vi "update hydrolysis feeding.vi"(7 "number_timestamps":i32, 8 "error in (no error)":errorcluster, 9 "amount":string, 10 "time":string, 11 "hydrolysis_specfile":string) -> (0 "error out":errorcluster)   [LabVIEW 2019, in "libFileFunctions.lvlib"]
doc: "void update_hydrolysis_feeding(const char* hydrolysis_specfile, double time[], double amount[], int number_timestamps);"
uses:
  libFileFunctions.lvlib
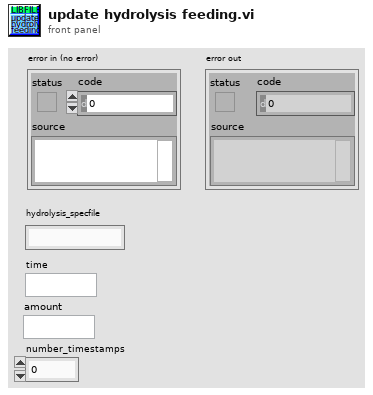
[diagram p1: front panel]
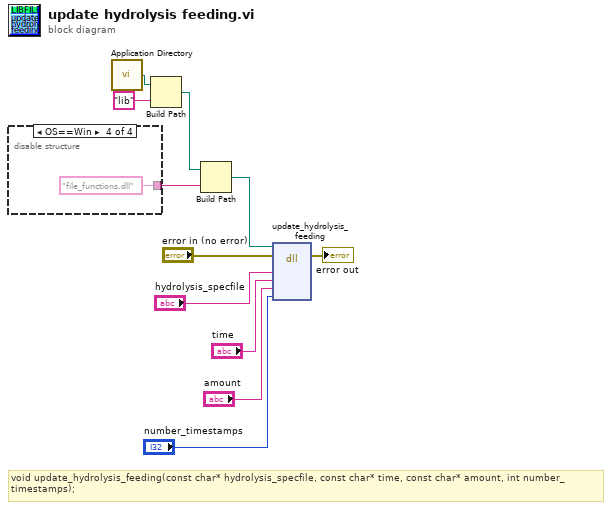
[diagram p0: block diagram]
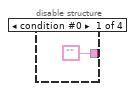
[diagram p2: hidden frame]
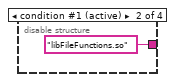
[diagram p3: hidden frame]
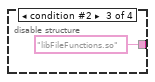
[diagram p4: hidden frame]
diagram:
  # "void update_hydrolysis_feeding(const char* hydrolysis_specfile, const char* time, const char* amount, int number_timestamps);"
  n1 = disable-structure shown="OS==Win" {
    disable-tunnel: ["" "libFileFunctions.so" ("name or relative path") "libFileFunctions.so" ("name or relative path") "file_functions.dll" ("name or relative path")] -> w2
    frame condition #0 {
    }
    frame condition #1 (active) {
    }
    frame condition #2 {
    }
    frame condition #3 {
    }
  }
  n2 = call <vilib>:"Application Directory.vi"() -> ("Application Directory"=w5:path)
  n3 = Build Path(base path=w5, name or relative path="lib") -> (appended path=w3:path)
  n4 = Build Path(base path=w3, name or relative path=w2) -> (appended path=w1:path)
  n5 = dll-call lib="home/paul/Schreibtisch/Biogas_plant_setup/LabView/lib/libFileFunctions/libFileFunctions.*" fn="update_hydrolysis_feeding"(path in=w1, error in="error in (no error)", "hydrolysis_specfile"="hydrolysis_specfile", "time"="time", "amount"="amount", "number_timestamps"="number_timestamps") -> (error out=→"error out":errorcluster)  [unwired: 6 in, 1 out]
